vi "Read_Values.vi"(7 "error in (no error)":errorcluster {"code" format="%.0x"}, 8 "Combo Box":string(combo), 9 "ChannelList":string, 10 "instrument handle out":refnum<k15>) -> (0 "error out":errorcluster, 2 "Val":dbl[][](array[numeric]), 3 "instrument handle 2":refnum<k15>)   [LabVIEW 2021]
uses:
  <instrlib>/Keysight DAQ970/Keysight DAQ970.lvlib
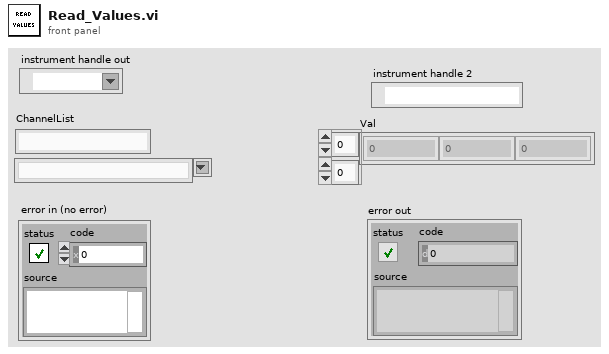
[diagram p1: front panel]
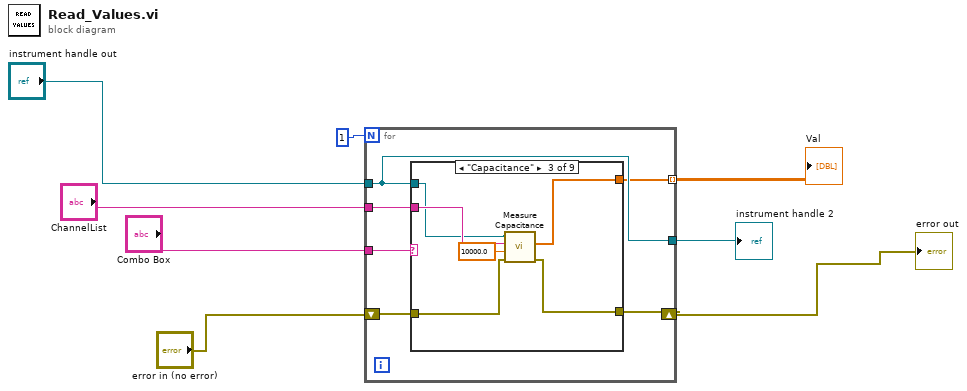
[diagram p0: block diagram]
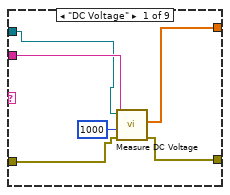
[diagram p2: hidden frame]
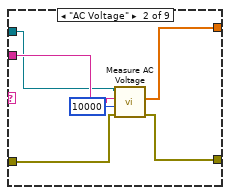
[diagram p3: hidden frame]
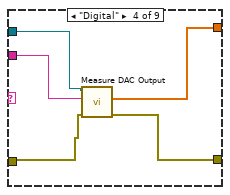
[diagram p4: hidden frame]
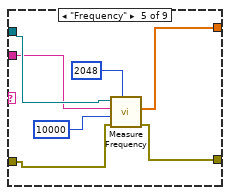
[diagram p5: hidden frame]
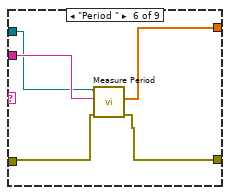
[diagram p6: hidden frame]
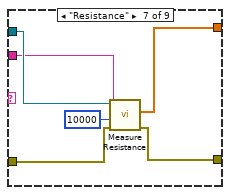
[diagram p7: hidden frame]
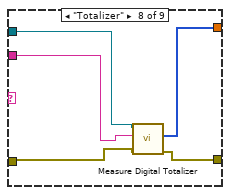
[diagram p8: hidden frame]
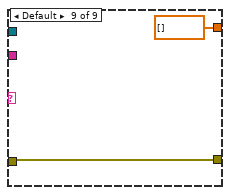
[diagram p9: hidden frame]
diagram:
  n1 = for {
    N: 1 -> [_]
    shift-right: [w14] -> w3
    shift-left: "error in (no error)" -> [w13]
    tunnel: "Combo Box" -> [w12]
    tunnel: "ChannelList" -> [w11]
    tunnel: "instrument handle out" -> [w10]
    tunnel: [w10] -> w7
    tunnel: [w9] -> w5 mode=indexing
    n2 = case shown="\"Capacitance\"" w12 {
      tunnel: [w18 w26 w29 w37 w41 w46 w52 w57 w62] -> w14
      tunnel: w13 -> [w19 w23 w28 w36 w42 w47 w53 w58 w62]
      tunnel: w11 -> [w20 w25 w32 w33 w43 w49 w54 w59 _]
      tunnel: w10 -> [w15 w24 w31 w34 w44 w48 w55 w60 _]
      tunnel: [w17 w22 w30 w35 w40 w45 w51 w56 dbl[] [] ("Val")] -> w9
      frame "DC Voltage" {
        n3 = call <instrlib>:"Measure DC Voltage.vi"("error in (no error)"=w19, "MaxTimeMilliseconds"=1000, "ChannelList"=w20, "instrument handle"=w15) -> ("error out"=w18:errorcluster, "Val"=w17:dbl[])  [unwired: 4 in, 2 out]
      }
      frame "AC Voltage" {
        n4 = call <instrlib>:"Measure AC Voltage.vi"("error in (no error)"=w23, "MaxTimeMilliseconds"=10000, "ChannelList"=w25, "instrument handle"=w24) -> ("error out"=w26:errorcluster, "Val"=w22:dbl[])  [unwired: 4 in, 2 out]
      }
      frame "Capacitance" {
        n5 = call <instrlib>:"Measure Capacitance.vi"("error in (no error)"=w28, "MaxTime"=10000.0, "ChannelList"=w32, "instrument handle"=w31) -> ("error out"=w29:errorcluster, "Val"=w30:dbl[])  [unwired: 4 in, 2 out]
      }
      frame "Digital" {
        n6 = call <instrlib>:"Measure DAC Output.vi"("error in (no error)"=w36, "ChannelList"=w33, "instrument handle"=w34) -> ("error out"=w37:errorcluster, "Val"=w35:dbl[])  [unwired: 5 in, 2 out]
      }
      frame "Frequency" {
        n7 = call <instrlib>:"Measure Frequency.vi"("ValBufferSize"=2048, "error in (no error)"=w42, "MaxTimeMilliseconds"=10000, "ChannelList"=w43, "instrument handle"=w44) -> ("error out"=w41:errorcluster, "Val"=w40:dbl[])  [unwired: 3 in, 2 out]
      }
      frame "Period " {
        n8 = call <instrlib>:"Measure Period.vi"("error in (no error)"=w47, "ChannelList"=w49, "instrument handle"=w48) -> ("error out"=w46:errorcluster, "Val"=w45:dbl[])  [unwired: 5 in, 2 out]
      }
      frame "Resistance" {
        n9 = call <instrlib>:"Measure Resistance.vi"("error in (no error)"=w53, "MaxTimeMilliseconds"=10000, "ChannelList"=w54, "instrument handle"=w55) -> ("error out"=w52:errorcluster, "Val"=w51:dbl[])  [unwired: 4 in, 2 out]
      }
      frame "Totalizer" {
        n10 = call <instrlib>:"Measure Digital Totalizer.vi"("error in (no error)"=w58, "ChannelList"=w59, "instrument handle"=w60) -> ("error out"=w57:errorcluster, "Val"=w56:i32[])  [unwired: 5 in, 2 out]
      }
      frame Default {
      }
    }
  }
  "error out" <- w3
  "Val" <- w5
  "instrument handle 2" <- w7
